vi "Save HTML to Text File.vi"() -> ()   [LabVIEW 2020]
uses:
  <vilib>/httpClient/LabVIEWHTTPClient.lvlib
panel:
  out "error out":errorcluster
  in  "Base Folder":path=path "C:/Personal/WPC Stat Scrape/Data/HTML Captures"
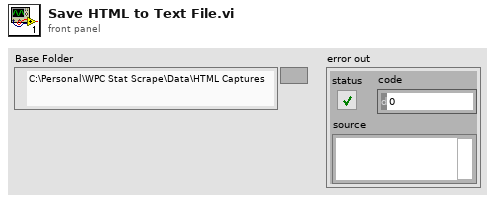
[diagram p1: front panel]
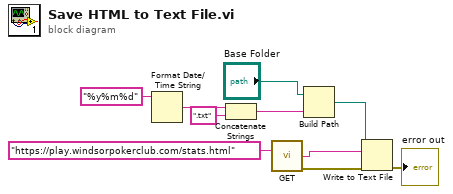
[diagram p0: block diagram]
diagram:
  n1 = Format Date/Time String(time format string (%c)="%y%m%d") -> (date/time string=w4:string)  [unwired: 2 in]
  n2 = Concatenate Strings(w4, ".txt" ("string")) -> (w2:string)
  n3 = call <vilib>:"GET.vi"("url"="https://play.windsorpokerclub.com/stats.html") -> ("body"=w9:string, "error out"=w8:errorcluster)  [unwired: 11 in, 2 out]
  n4 = Build Path(base path="Base Folder", name or relative path=w2) -> (appended path=w3:path)
  n5 = Write to Text File(file (use dialog)=w3, text=w9, error in=w8) -> (error out=→"error out":errorcluster)  [unwired: 1 in, 2 out]
